vi "BRig_RT__Case_Exp__State_initTrial.vi"(0 "input_dataCurrent":u16[](array[numeric]), 9 "input_dataBlock":u16[][](array[numeric]), 11 "input_dataTrial":u16[][](array[numeric]), 12 "input_dataExp":u16[](array[numeric])) -> (1 "output_iTrial":u16, 2 "output_nTrial":u16, 3 "output_SolenoidReward":bool, 4 "output_dataCurrent":u16[](array[numeric]), 10 "output_dataBlock":u16[][](array[numeric]), 15 "output_dataTrial":u16[][](array[numeric]))   [LabVIEW 2014]
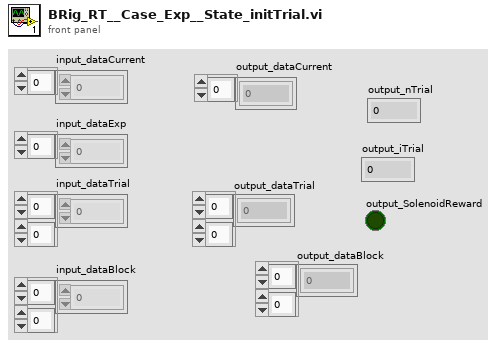
[diagram p1: front panel]
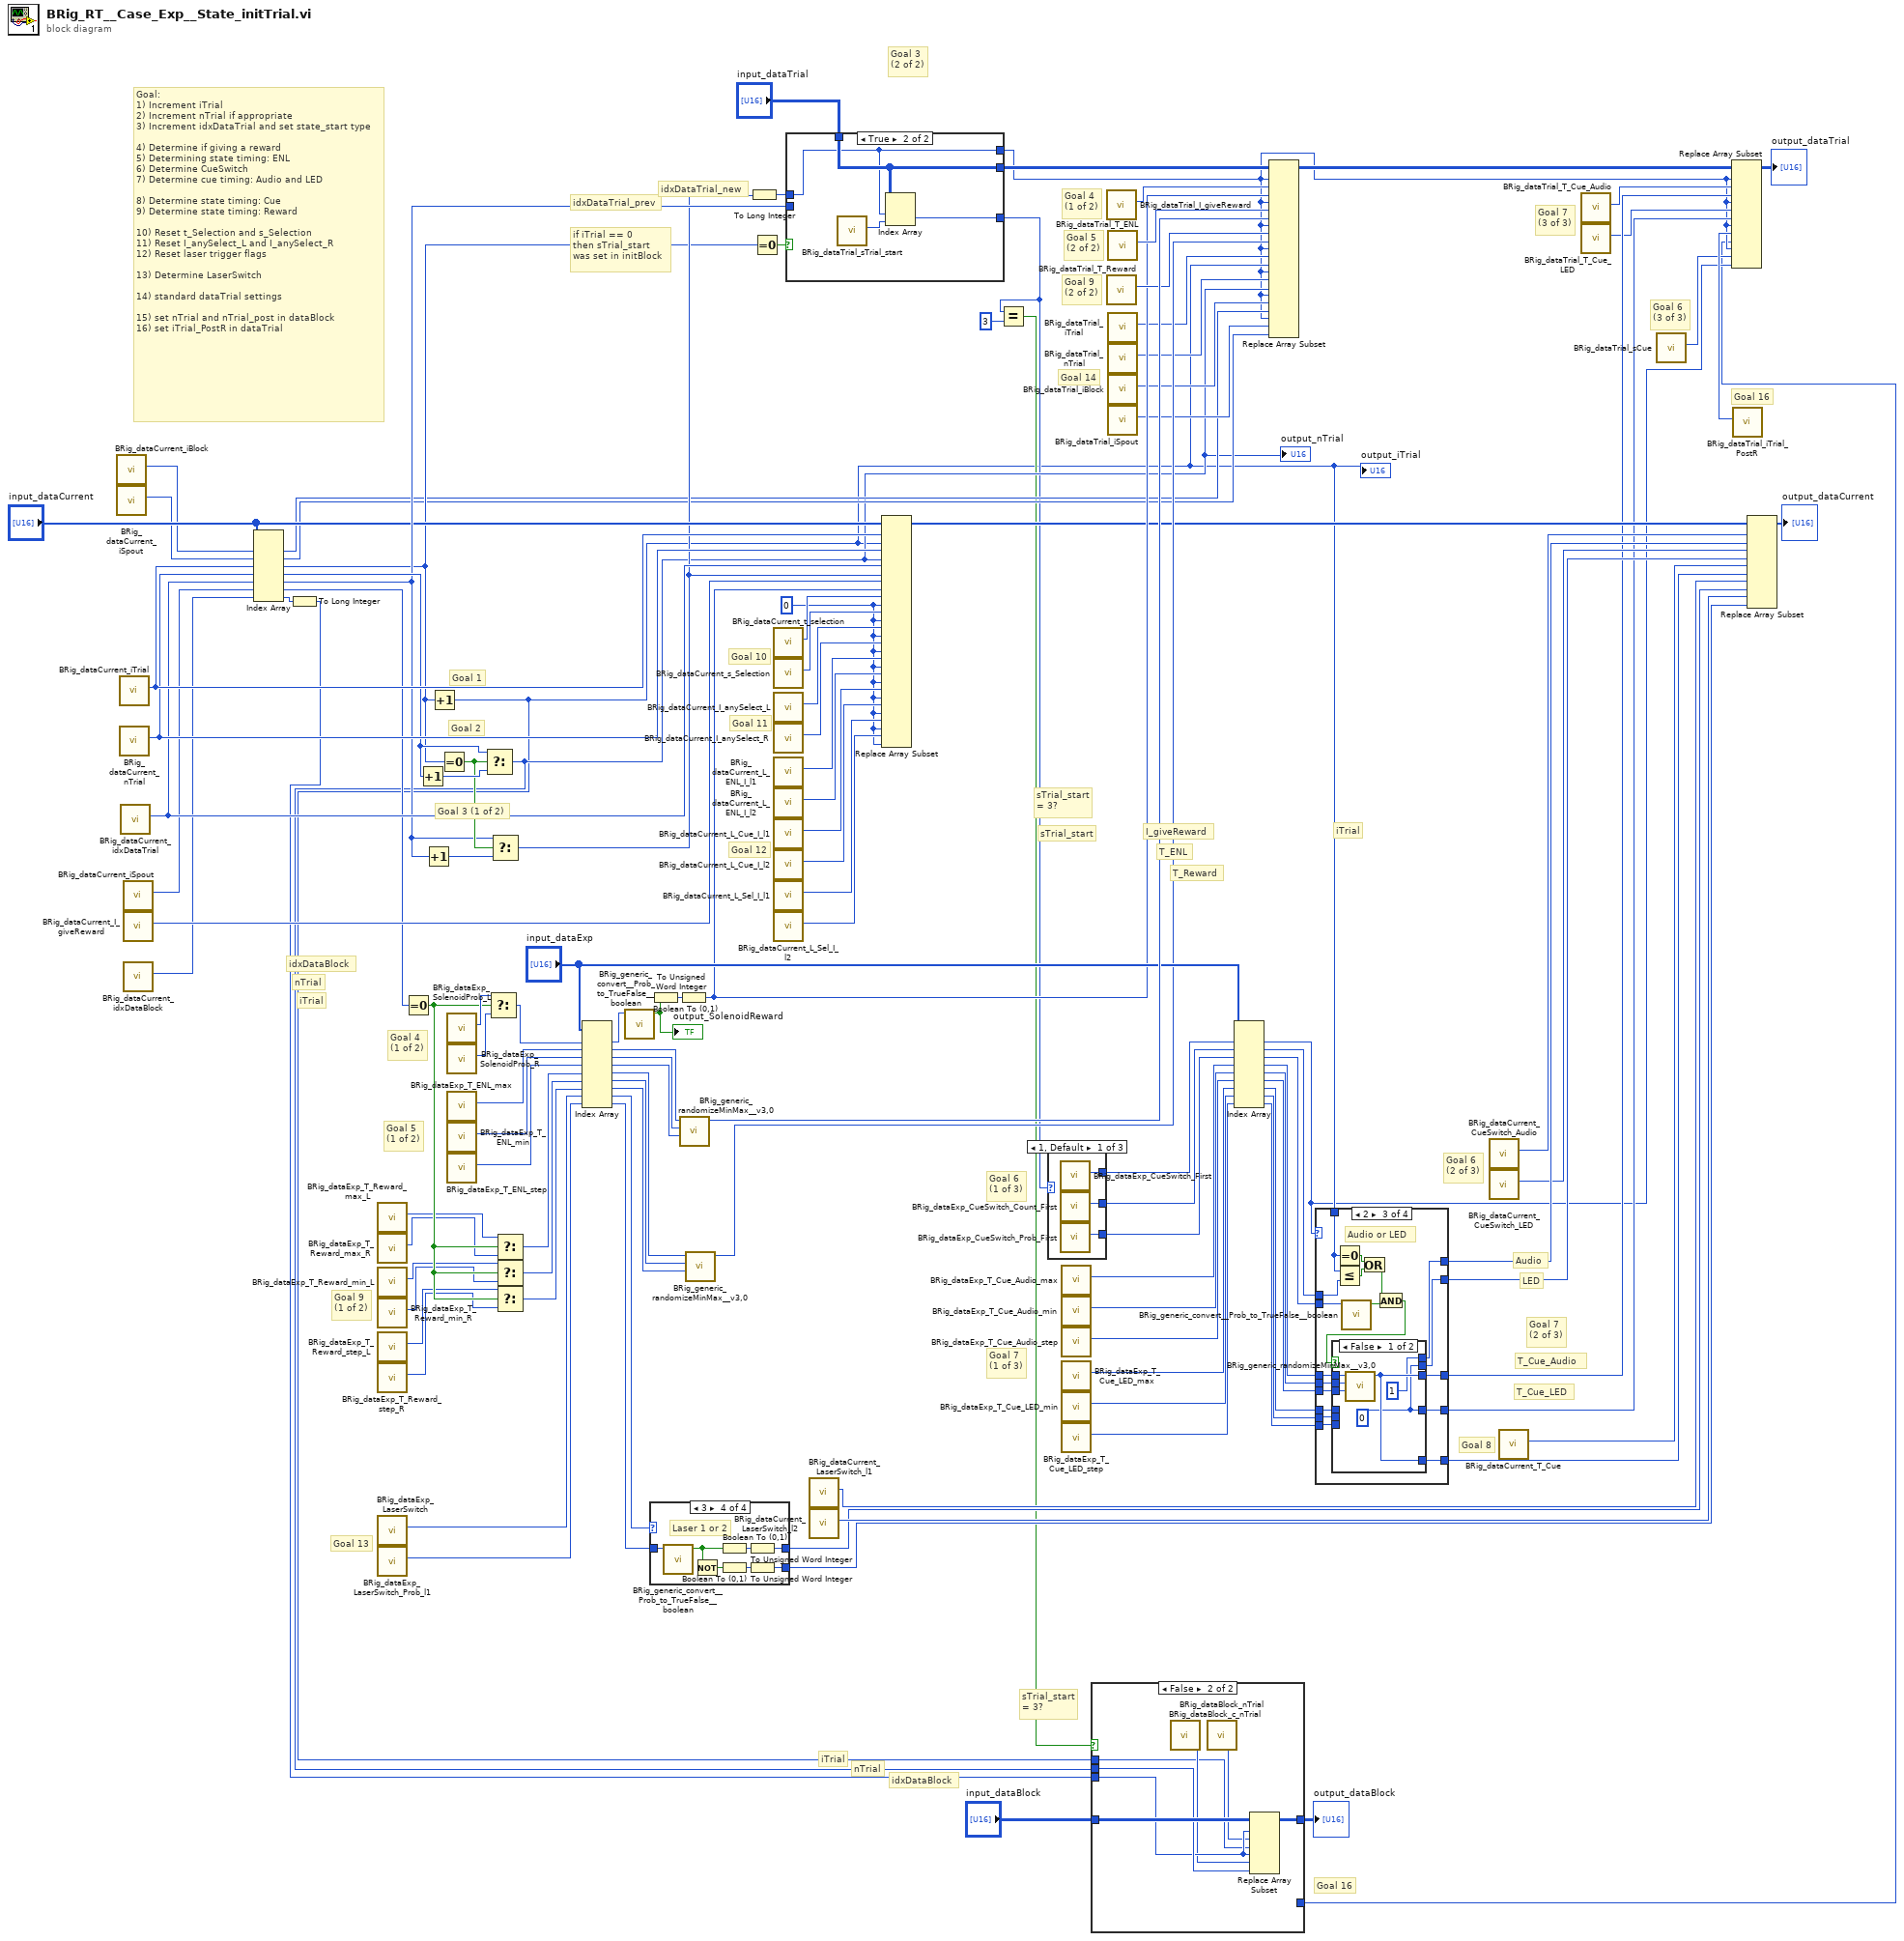
[diagram p0: block diagram]
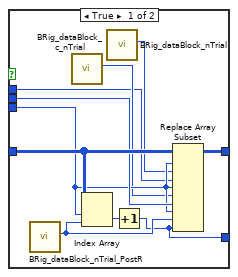
[diagram p2: hidden frame]
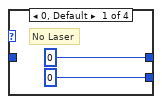
[diagram p3: hidden frame]
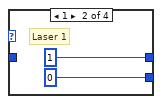
[diagram p4: hidden frame]
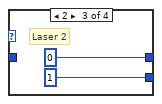
[diagram p5: hidden frame]
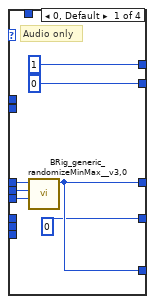
[diagram p6: hidden frame]
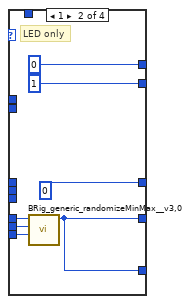
[diagram p7: hidden frame]
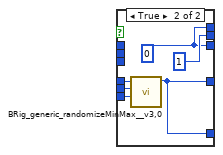
[diagram p8: hidden frame]
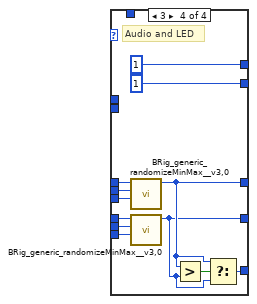
[diagram p9: hidden frame]
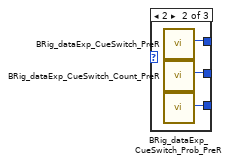
[diagram p10: hidden frame]
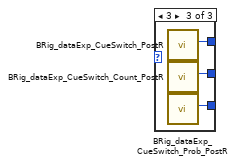
[diagram p11: hidden frame]
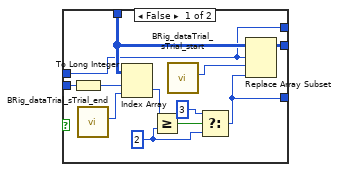
[diagram p12: hidden frame]
diagram:
  w73 = u16 0 ("new element/subarray")
  # "Goal 16"
  # "Goal 6\n(3 of 3)"
  # "iTrial"
  # "iTrial"
  # "Goal 16"
  # "sTrial_start\n= 3?"
  # "sTrial_start\n= 3?"
  # "idxDataBlock"
  # "nTrial"
  # "idxDataBlock"
  # "nTrial"
  # "Goal 14"
  # "Goal 13"
  # "iTrial"
  # "Goal 8"
  # "Goal 7\n(3 of 3)"
  # "Goal 7\n(2 of 3)"
  # "Goal 7\n(1 of 3)"
  # "T_Cue_LED"
  # "T_Cue_Audio"
  # "I_giveReward"
  # "Goal 4\n(1 of 2)"
  # "T_Reward"
  # "Goal 9\n(2 of 2)"
  # "Goal 9\n(1 of 2)"
  # "Goal 12"
  # "Goal 11"
  # "Goal 10"
  # "T_ENL"
  # "sTrial_start"
  # "LED"
  # "Audio"
  # "Goal 6\n(2 of 3)"
  # "Goal 6\n(1 of 3)"
  # "Goal 3\n(2 of 2)"
  # "Goal 5\n(2 of 2)"
  # "idxDataTrial_new"
  # "Goal 5\n(1 of 2)"
  # "Goal 4\n(1 of 2)"
  # "idxDataTrial_prev"
  # "if iTrial == 0\nthen sTrial_start\nwas set in initBlock"
  # "Goal 3 (1 of 2)"
  # "Goal 2"
  # "Goal 1"
  # "Goal:\n1) Increment iTrial\n2) Increment nTrial if appropriate\n3) Increment idxDataTrial and set state_start type\n\n4) Determine if giving a reward\n5) Determining state timing: ENL\n6) Determine CueSwitch\n7) Determine cue timing: Audio and LED\n\n8) Determine state timing: Cue\n9) Determine state timing: Reward\n\n10) Reset t_Selection and s_Selection\n11) Reset I_anySelect_L and I_anySelect_R\n12) Reset laser trigger flags\n\n13) Determine LaserSwitch\n\n14) standard dataTrial settings\n\n15) set nTrial and nTrial_post in dataBlock\n16) set iTrial_PostR in dataTrial"
  n1 = call "BRig_dataCurrent_iBlock.vi"() -> ("output_iBlock"=w6:i32)  [unwired: 11 in]
  n2 = call "BRig_dataCurrent_iSpout.vi"() -> ("output_iSpout"=w5:i32)  [unwired: 11 in]
  n3 = call "BRig_dataCurrent_iTrial.vi"() -> ("output_iTrial"=w122:i32)  [unwired: 11 in]
  n4 = call "BRig_dataCurrent_nTrial.vi"() -> ("output_nTrial"=w121:i32)  [unwired: 11 in]
  n5 = call "BRig_dataCurrent_idxDataTrial.vi"() -> ("output_idxDataTrial"=w118:i32)  [unwired: 11 in]
  n6 = call "BRig_dataCurrent_iSpout.vi"() -> ("output_iSpout"=w111:i32)  [unwired: 11 in]
  n7 = call "BRig_dataCurrent_I_giveReward.vi"() -> ("output_I_giveReward"=w110:i32)  [unwired: 11 in]
  n8 = call "BRig_dataCurrent_idxDataBlock.vi"() -> ("output_idxDataBlock"=w23:i32)  [unwired: 11 in]
  n9 = Index Array(array="input_dataCurrent", index #1=w6, index #2=w5, index #3=w122, index #4=w121, index #5=w118, index #6=w111, index #7=w23) -> (element #1=w25:u16, element #2=w24:u16, element #3=w38:u16, element #4=w120:u16, element #5=w113:u16, element #6=w109:u16, element #7=w20:u16)
  n10 = To Long Integer(number=w20) -> (32bit integer=w19:i32)
  n11 = call "BRig_dataExp_T_Reward_max_L.vi"() -> ("output_T_Reward_max_L"=w71:i32)  [unwired: 11 in]
  n12 = call "BRig_dataExp_T_Reward_max_R.vi"() -> ("output_T_Reward_max_R"=w70:i32)  [unwired: 11 in]
  n13 = call "BRig_dataExp_T_Reward_min_L.vi"() -> ("output_Tcycle_Reward_min_L"=w69:i32)  [unwired: 11 in]
  n14 = call "BRig_dataExp_T_Reward_min_R.vi"() -> ("output_T_Reward_min_R"=w68:i32)  [unwired: 11 in]
  n15 = call "BRig_dataExp_T_Reward_step_L.vi"() -> ("output_T_Reward_step_L"=w67:i32)  [unwired: 11 in]
  n16 = call "BRig_dataExp_T_Reward_step_R.vi"() -> ("output_T_Reward_step_R"=w66:i32)  [unwired: 11 in]
  n17 = call "BRig_dataExp_LaserSwitch.vi"() -> ("output_LaserSwitch"=w37:i32)  [unwired: 11 in]
  n18 = call "BRig_dataExp_LaserSwitch_Prob_l1.vi"() -> ("output_LaserSwitch_Probability_L1"=w36:i32)  [unwired: 11 in]
  n19 = Equal To 0?(x=w109) -> (x = 0?=w72:bool)
  n20 = Increment(x=w120) -> (x+1=w119:u16)
  n21 = Increment(x=w113) -> (x+1=w116:u16)
  n22 = Increment(x=w38) -> (x+1=w7:u16)
  "output_iTrial" <- w7
  n23 = Equal To 0?(x=w38) -> (x = 0?=w117:bool)
  n24 = call "BRig_dataExp_SolenoidProb_L.vi"() -> ("output_SolenoidProbability_L"=w108:i32)  [unwired: 11 in]
  n25 = call "BRig_dataExp_SolenoidProb_R.vi"() -> ("output_SolenoidProbability_R"=w107:i32)  [unwired: 11 in]
  n26 = call "BRig_dataExp_T_ENL_max.vi"() -> ("output_T_ENL_max"=w101:i32)  [unwired: 11 in]
  n27 = call "BRig_dataExp_T_ENL_min.vi"() -> ("output_T_ENL_min"=w102:i32)  [unwired: 11 in]
  n28 = call "BRig_dataExp_T_ENL_step.vi"() -> ("output_T_ENL_step"=w103:i32)  [unwired: 11 in]
  n29 = Select(t=w120, s=w117, f=w119) -> (s? t:f=w21:u16)
  "output_nTrial" <- w21
  n30 = Select(t=w108, s=w72, f=w107) -> (s? t:f=w106:i32)
  n31 = Select(t=w113, s=w117, f=w116) -> (s? t:f=w97:u16)
  n32 = Select(t=w71, s=w72, f=w70) -> (s? t:f=w65:i32)
  n33 = Select(t=w69, s=w72, f=w68) -> (s? t:f=w64:i32)
  n34 = Select(t=w67, s=w72, f=w66) -> (s? t:f=w63:i32)
  n35 = Index Array(array="input_dataExp", index #1=w106, index #2=w101, index #3=w102, index #4=w103, index #5=w65, index #6=w64, index #7=w63, index #8=w37, index #9=w36) -> (element #1=w105:u16, element #2=w100:u16, element #3=w99:u16, element #4=w98:u16, element #5=w62:u16, element #6=w61:u16, element #7=w60:u16, element #8=w35:u16, element #9=w34:u16)
  n36 = call "BRig_generic_convert__Prob_to_TrueFalse__boolean.vi"("input_probability_u16"=w105) -> ("output_TF"=w104:bool)  [unwired: 10 in]
  "output_SolenoidReward" <- w104
  n37 = case shown="3" w35 {
    tunnel: [u16 0 u16 1 u16 0 w133] -> w32
    tunnel: [u16 0 u16 0 u16 1 w130] -> w31
    tunnel: w34 -> [_ _ _ w136]
    frame 0, Default {
      # "No Laser"
    }
    frame 1 {
      # "Laser 1"
    }
    frame 2 {
      # "Laser 2"
    }
    frame 3 {
      # "Laser 1 or 2"
      n38 = call "BRig_generic_convert__Prob_to_TrueFalse__boolean.vi"("input_probability_u16"=w136) -> ("output_TF"=w132:bool)  [unwired: 10 in]
      n39 = Not(x=w132) -> (.not. x?=w131:bool)
      n40 = Boolean To (0,1)(Boolean=w132) -> (0, 1=w134:i16)
      n41 = Boolean To (0,1)(Boolean=w131) -> (0, 1=w135:i16)
      n42 = To Unsigned Word Integer(number=w134) -> (unsigned 16bit integer=w133:u16)
      n43 = To Unsigned Word Integer(number=w135) -> (unsigned 16bit integer=w130:u16)
    }
  }
  n44 = Boolean To (0,1)(Boolean=w104) -> (0, 1=w123:i16)
  n45 = To Unsigned Word Integer(number=w123) -> (unsigned 16bit integer=w56:u16)
  n46 = call "BRig_generic_randomizeMinMax__v3,0.vi"("Input_Increment"=w98, "Input_Min"=w99, "Input_Max"=w100) -> ("Output"=w93:u16)  [unwired: 8 in]
  n47 = call "BRig_generic_randomizeMinMax__v3,0.vi"("Input_Increment"=w60, "Input_Min"=w61, "Input_Max"=w62) -> ("Output"=w58:u16)  [unwired: 8 in]
  n48 = To Long Integer(number=w97) -> (32bit integer=w96:i32)
  n49 = Equal To 0?(x=w38) -> (x = 0?=w115:bool)
  n50 = call "BRig_dataCurrent_t_selection.vi"() -> ("output_t_selection"=w83:i32)  [unwired: 11 in]
  n51 = call "BRig_dataCurrent_s_Selection.vi"() -> ("output_s_Selection"=w82:i32)  [unwired: 11 in]
  n52 = call "BRig_dataCurrent_I_anySelect_L.vi"() -> ("output_IanySelect_L"=w81:i32)  [unwired: 11 in]
  n53 = call "BRig_dataCurrent_I_anySelect_R.vi"() -> ("output_IanySelect_R"=w80:i32)  [unwired: 11 in]
  n54 = call "BRig_dataCurrent_L_ENL_I_l1.vi"() -> ("output_L_ENL_I_l1"=w79:i32)  [unwired: 11 in]
  n55 = call "BRig_dataCurrent_L_ENL_I_l2.vi"() -> ("output_L_ENL_I_l2"=w78:i32)  [unwired: 11 in]
  n56 = call "BRig_dataCurrent_L_Cue_I_l1.vi"() -> ("output_L_Cue_I_l1"=w77:i32)  [unwired: 11 in]
  n57 = call "BRig_dataCurrent_L_Cue_I_l2.vi"() -> ("output_L_Cue_I_l2"=w76:i32)  [unwired: 11 in]
  n58 = call "BRig_dataCurrent_L_Sel_I_l1.vi"() -> ("output_L_Sel_I_l1"=w75:i32)  [unwired: 11 in]
  n59 = call "BRig_dataCurrent_L_Sel_I_l2.vi"() -> ("output_L_Sel_I_l2"=w74:i32)  [unwired: 11 in]
  n60 = case shown="True" w115 {
    tunnel: "input_dataTrial" -> [w145 w152]
    tunnel: [w144 w152] -> w95
    tunnel: w113 -> [w148 _]
    tunnel: w96 -> [w137 w151]
    tunnel: [w137 w151] -> w4
    tunnel: [w139 w149] -> w14
    frame False {
      w140 = u16 2 ("y")
      n61 = To Long Integer(number=w148) -> (32bit integer=w143:i32)
      n62 = call "BRig_dataTrial_sTrial_end.vi"() -> ("output_sTrial_end"=w147:i32)  [unwired: 11 in]
      n63 = Index Array(array=w145, index (row)=w143, index (col)=w147) -> (element=w146:u16)
      n64 = Greater Or Equal?(x=w146, y=w140) -> (x >= y?=w142:bool)
      n65 = call "BRig_dataTrial_sTrial_start.vi"() -> ("output_sTrial_start"=w138:i32)  [unwired: 11 in]
      n66 = Select(t=u16 3 ("y"), s=w142, f=w140) -> (s? t:f=w139:u16)
      n67 = Replace Array Subset(array=w145, new element=w139, index (row)=w137, index (col)=w138) -> (w144:u16[][])
    }
    frame True {
      n68 = call "BRig_dataTrial_sTrial_start.vi"() -> ("output_sTrial_start"=w150:i32)  [unwired: 11 in]
      n69 = Index Array(array=w152, index (row)=w151, index (col)=w150) -> (element=w149:u16)
    }
  }
  n70 = call "BRig_dataCurrent_LaserSwitch_l1.vi"() -> ("output_LaserSwitch_l1"=w30:i32)  [unwired: 11 in]
  n71 = call "BRig_dataCurrent_LaserSwitch_l2.vi"() -> ("output_LaserSwitch_l2"=w33:i32)  [unwired: 11 in]
  n72 = Replace Array Subset(array="input_dataCurrent", new element #1=w7, index #1=w122, new element #2=w21, index #2=w121, new element #3=w97, index #3=w118, new element #4=w56, index #4=w110, new element #5=w73, index #5=w83, new element #6=w73, index #6=w82, new element #7=w73, index #7=w81, new element #8=w73, index #8=w80, new element #9=w73, index #9=w79, new element #10=w73, index #10=w78, new element #11=w73, index #11=w77, new element #12=w73, index #12=w76, new element #13=w73, index #13=w75, new element #14=w73, index #14=w74) -> (w17:u16[])
  n73 = Equal?(x=w14, y=u16 3) -> (x = y?=w13:bool)
  n74 = case shown="1, Default" w14 {
    tunnel: [w155 w156 w161] -> w90
    tunnel: [w154 w157 w160] -> w89
    tunnel: [w153 w158 w159] -> w88
    frame 1, Default {
      n75 = call "BRig_dataExp_CueSwitch_First.vi"() -> ("output_CueSwitch_First"=w155:i32)  [unwired: 11 in]
      n76 = call "BRig_dataExp_CueSwitch_Count_First.vi"() -> ("output_CueSwitch_Count_First"=w154:i32)  [unwired: 11 in]
      n77 = call "BRig_dataExp_CueSwitch_Prob_First.vi"() -> ("output_CueSwitch_Prob_First"=w153:i32)  [unwired: 11 in]
    }
    frame 2 {
      n78 = call "BRig_dataExp_CueSwitch_PreR.vi"() -> ("output_CueSwitch_PreR"=w156:i32)  [unwired: 11 in]
      n79 = call "BRig_dataExp_CueSwitch_Count_PreR.vi"() -> ("output_CueSwitch_Count_PreR"=w157:i32)  [unwired: 11 in]
      n80 = call "BRig_dataExp_CueSwitch_Prob_PreR.vi"() -> ("output_CueSwitch_Prob_PreR"=w158:i32)  [unwired: 11 in]
    }
    frame 3 {
      n81 = call "BRig_dataExp_CueSwitch_PostR.vi"() -> ("output_CueSwitch_PostR"=w161:i32)  [unwired: 11 in]
      n82 = call "BRig_dataExp_CueSwitch_Count_PostR.vi"() -> ("output_CueSwitch_Count_PostR"=w160:i32)  [unwired: 11 in]
      n83 = call "BRig_dataExp_CueSwitch_Prob_PostR.vi"() -> ("output_CueSwitch_Prob_PostR"=w159:i32)  [unwired: 11 in]
    }
  }
  n84 = call "BRig_dataExp_T_Cue_Audio_max.vi"() -> ("output_T_Cue_Audio_max"=w55:i32)  [unwired: 11 in]
  n85 = call "BRig_dataExp_T_Cue_Audio_min.vi"() -> ("output_T_Cue_Audio_min"=w54:i32)  [unwired: 11 in]
  n86 = call "BRig_dataExp_T_Cue_Audio_step.vi"() -> ("output_T_Cue_Audio_step"=w53:i32)  [unwired: 11 in]
  n87 = call "BRig_dataExp_T_Cue_LED_max.vi"() -> ("output_T_Cue_LED_max"=w52:i32)  [unwired: 11 in]
  n88 = call "BRig_dataExp_T_Cue_LED_min.vi"() -> ("output_T_Cue_LED_min"=w51:i32)  [unwired: 11 in]
  n89 = call "BRig_dataExp_T_Cue_LED_step.vi"() -> ("output_T_Cue_LED_step"=w50:i32)  [unwired: 11 in]
  n90 = case shown="False" w13 {
    tunnel: w21 -> [w168 w177]
    tunnel: "input_dataBlock" -> [w171 w178]
    tunnel: w19 -> [w166 w175]
    tunnel: [w167 w176] -> w18
    tunnel: w7 -> [w163 w172]
    tunnel: [w162 _] -> w1
    frame True {
      n91 = call "BRig_dataBlock_nTrial_PostR.vi"() -> ("output_nTrial_PostR"=w170:i32)  [unwired: 11 in]
      n92 = call "BRig_dataBlock_c_nTrial.vi"() -> ("output_c_nTrial"=w165:i32)  [unwired: 11 in]
      n93 = Index Array(array=w171, index (row)=w166, index (col)=w170) -> (element=w169:u16)
      n94 = call "BRig_dataBlock_nTrial.vi"() -> ("output_nTrial"=w164:i32)  [unwired: 11 in]
      n95 = Increment(x=w169) -> (x+1=w162:u16)
      n96 = Replace Array Subset(array=w171, new element #1=w163, index (row) #1=w166, index (col) #1=w164, new element #2=w168, index (row) #2=w166, index (col) #2=w165, new element #3=w162, index (row) #3=w166, index (col) #3=w170) -> (w167:u16[][])
    }
    frame False {
      n97 = call "BRig_dataBlock_c_nTrial.vi"() -> ("output_c_nTrial"=w173:i32)  [unwired: 11 in]
      n98 = call "BRig_dataBlock_nTrial.vi"() -> ("output_nTrial"=w174:i32)  [unwired: 11 in]
      n99 = Replace Array Subset(array=w178, new element #1=w172, index (row) #1=w175, index (col) #1=w174, new element #2=w177, index (row) #2=w175, index (col) #2=w173) -> (w176:u16[][])
    }
  }
  "output_dataBlock" <- w18
  n100 = call "BRig_dataTrial_I_giveReward.vi"() -> ("output_I_giveReward"=w57:i32)  [unwired: 11 in]
  n101 = call "BRig_dataTrial_T_Reward.vi"() -> ("output_T_Reward"=w59:i32)  [unwired: 11 in]
  n102 = call "BRig_dataTrial_T_ENL.vi"() -> ("output_T_ENL"=w94:i32)  [unwired: 11 in]
  n103 = call "BRig_dataTrial_iTrial.vi"() -> ("output_iTrial"=w29:i32)  [unwired: 11 in]
  n104 = call "BRig_dataTrial_nTrial.vi"() -> ("output_nTrial"=w28:i32)  [unwired: 11 in]
  n105 = call "BRig_dataTrial_iBlock.vi"() -> ("output_iBlock"=w27:i32)  [unwired: 11 in]
  n106 = call "BRig_dataTrial_iSpout.vi"() -> ("output_iSpout"=w26:i32)  [unwired: 11 in]
  n107 = Index Array(array="input_dataExp", index #1=w90, index #2=w89, index #3=w88, index #4=w55, index #5=w54, index #6=w53, index #7=w52, index #8=w51, index #9=w50) -> (element #1=w2:u16, element #2=w49:u16, element #3=w48:u16, element #4=w47:u16, element #5=w46:u16, element #6=w45:u16, element #7=w44:u16, element #8=w43:u16, element #9=w42:u16)
  n108 = Replace Array Subset(array=w95, new element #1=w56, index (row) #1=w4, index (col) #1=w57, new element #2=w93, index (row) #2=w4, index (col) #2=w94, new element #3=w58, index (row) #3=w4, index (col) #3=w59, new element #4=w7, index (row) #4=w4, index (col) #4=w29, new element #5=w21, index (row) #5=w4, index (col) #5=w28, new element #6=w25, index (row) #6=w4, index (col) #6=w27, new element #7=w24, index (row) #7=w4, index (col) #7=w26) -> (w16:u16[][])
  n109 = case shown="2" w2 {
    tunnel: [u16 1 u16 0 w197 u16 1] -> w86
    tunnel: [u16 0 u16 1 w196 u16 1] -> w84
    tunnel: w49 -> [_ _ w210 _]
    tunnel: w48 -> [_ _ w207 _]
    tunnel: w47 -> [w183 _ w203 w233]
    tunnel: w46 -> [w182 _ w202 w232]
    tunnel: w45 -> [w181 _ w201 w231]
    tunnel: w44 -> [_ w190 w195 w230]
    tunnel: w43 -> [_ w189 w194 w229]
    tunnel: w42 -> [_ w188 w193 w228]
    tunnel: [w180 u16 0 ("Output") w200 w226] -> w11
    tunnel: [u16 0 ("Output") w187 w198 w225] -> w10
    tunnel: [w180 w187 w199 w224] -> w39
    tunnel: w7 -> [_ _ w211 _]
    frame 0, Default {
      # "Audio only"
      n110 = call "BRig_generic_randomizeMinMax__v3,0.vi"("Input_Increment"=w181, "Input_Min"=w182, "Input_Max"=w183) -> ("Output"=w180:u16)  [unwired: 8 in]
    }
    frame 1 {
      # "LED only"
      n111 = call "BRig_generic_randomizeMinMax__v3,0.vi"("Input_Increment"=w188, "Input_Min"=w189, "Input_Max"=w190) -> ("Output"=w187:u16)  [unwired: 8 in]
    }
    frame 2 {
      # "Audio or LED"
      n112 = Equal To 0?(x=w211) -> (x = 0?=w209:bool)
      n113 = Less Or Equal?(x=w211, y=w210) -> (x <= y?=w208:bool)
      n114 = call "BRig_generic_convert__Prob_to_TrueFalse__boolean.vi"("input_probability_u16"=w207) -> ("output_TF"=w206:bool)  [unwired: 10 in]
      n115 = Or(x=w209, y=w208) -> (x .or. y?=w205:bool)
      n116 = And(x=w205, y=w206) -> (x .and. y?=w204:bool)
      n117 = case shown="False" w204 {
        tunnel: w203 -> [w217 _]
        tunnel: w202 -> [w216 _]
        tunnel: w201 -> [w215 _]
        tunnel: [w214 w218] -> w200
        tunnel: [w214 w220] -> w199
        tunnel: [w212 w220] -> w198
        tunnel: [u16 1 w218] -> w197
        tunnel: [w212 u16 1] -> w196
        tunnel: w195 -> [_ w223]
        tunnel: w194 -> [_ w222]
        tunnel: w193 -> [_ w221]
        frame False {
          w212 = u16 0
          n118 = call "BRig_generic_randomizeMinMax__v3,0.vi"("Input_Increment"=w215, "Input_Min"=w216, "Input_Max"=w217) -> ("Output"=w214:u16)  [unwired: 8 in]
        }
        frame True {
          w218 = u16 0
          n119 = call "BRig_generic_randomizeMinMax__v3,0.vi"("Input_Increment"=w221, "Input_Min"=w222, "Input_Max"=w223) -> ("Output"=w220:u16)  [unwired: 8 in]
        }
      }
    }
    frame 3 {
      # "Audio and LED"
      n120 = call "BRig_generic_randomizeMinMax__v3,0.vi"("Input_Increment"=w231, "Input_Min"=w232, "Input_Max"=w233) -> ("Output"=w226:u16)  [unwired: 8 in]
      n121 = call "BRig_generic_randomizeMinMax__v3,0.vi"("Input_Increment"=w228, "Input_Min"=w229, "Input_Max"=w230) -> ("Output"=w225:u16)  [unwired: 8 in]
      n122 = Greater?(x=w226, y=w225) -> (0:w227:bool)
      n123 = Select(t=w226, s=w227, f=w225) -> (s? t:f=w224:u16)
    }
  }
  n124 = call "BRig_dataCurrent_CueSwitch_Audio.vi"() -> ("output_CueSwitch_Audio"=w87:i32)  [unwired: 11 in]
  n125 = call "BRig_dataCurrent_CueSwitch_LED.vi"() -> ("output_CueSwitch_LED"=w85:i32)  [unwired: 11 in]
  n126 = call "BRig_dataCurrent_T_Cue.vi"() -> ("output_T_Cue"=w40:i32)  [unwired: 11 in]
  n127 = call "BRig_dataTrial_T_Cue_Audio.vi"() -> ("output_T_Cue_Audio"=w9:i32)  [unwired: 11 in]
  n128 = call "BRig_dataTrial_T_Cue_LED.vi"() -> ("output_T_Cue_LED"=w8:i32)  [unwired: 11 in]
  n129 = call "BRig_dataTrial_sCue.vi"() -> ("output_sCue"=w3:i32)  [unwired: 11 in]
  n130 = call "BRig_dataTrial_iTrial_PostR.vi"() -> ("output_iTrial_PostR"=w12:i32)  [unwired: 11 in]
  n131 = Replace Array Subset(array=w16, new element #1=w11, index (row) #1=w4, index (col) #1=w9, new element #2=w10, index (row) #2=w4, index (col) #2=w8, new element #3=w1, index (row) #3=w4, index (col) #3=w12, new element #4=w2, index (row) #4=w4, index (col) #4=w3) -> (→"output_dataTrial":u16[][])
  n132 = Replace Array Subset(array=w17, new element #1=w86, index #1=w87, new element #2=w84, index #2=w85, new element #3=w39, index #3=w40, new element #4=w32, index #4=w30, new element #5=w31, index #5=w33) -> (→"output_dataCurrent":u16[])
